vi "SubVI_Overlay Circle Result.vi"(7 "Overlay Result":bool, 8 "Max & min":T2 {"Min Position"."Y" format="%.2f"; "Min Position"."X" format="%.2f"; "Max Position"."Y" format="%.2f"; "Max Position"."X" format="%.2f"}, 9 "Result":cluster{"Name":string, "NG?":bool, "Score":dbl}, 10 "Result In":T3 {"Center"."Y" format="%.2f"; "Center"."X" format="%.2f"}, 11 "Image":T1) -> ()   [LabVIEW 2013]
uses:
  <vilib>/vision/Image Controls.llb/IMAQ Image.ctl
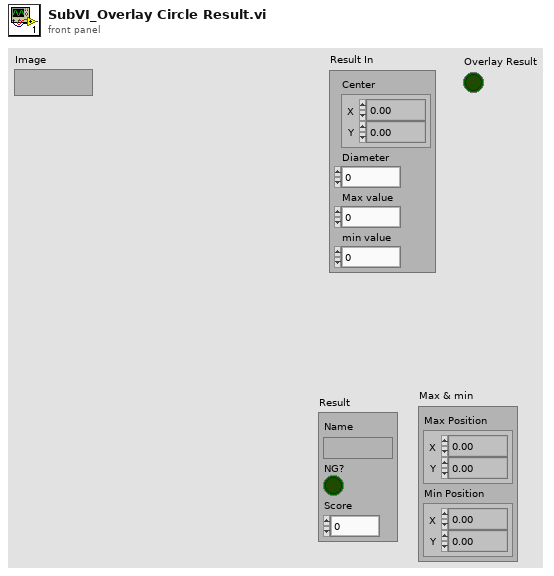
[diagram p1: front panel]
types:
  T1 = typedef "IMAQ Image.ctl" = refnum<image>
  T2 = cluster{"Max Position":cluster{"X":sgl, "Y":sgl}, "Min Position":cluster{"X":sgl, "Y":sgl}}
  T3 = cluster{"Center":cluster{"X":sgl, "Y":sgl}, "Diameter":dbl, "Max value":sgl, "min value":sgl}
  T4 = cluster{"Max Position":cluster{"X":i32, "Y":i32}, "Min Position":cluster{"X":i32, "Y":i32}}
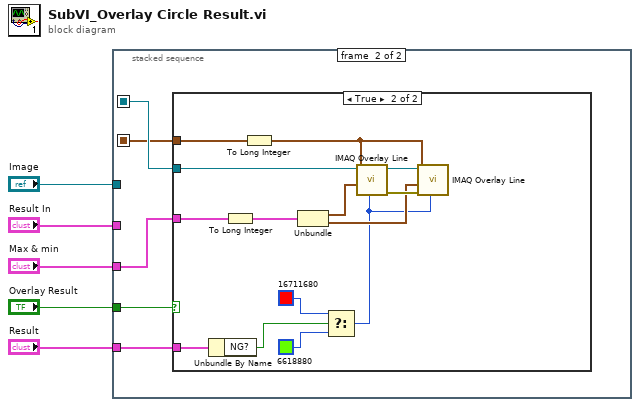
[diagram p0: block diagram]
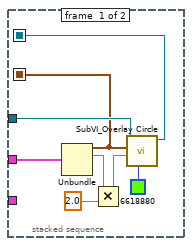
[diagram p2: hidden frame]
diagram:
  n1 = stacked-sequence {
    seq-local: [w10 _] -> [_ w16]
    seq-local: [w9 _] -> [_ w15]
    tunnel: "Image" -> [w11 _]
    tunnel: "Result In" -> [w12 _]
    tunnel: "Max & min" -> [_ w17]
    tunnel: "Overlay Result" -> [_ w18]
    tunnel: "Result" -> [_ w14]
    frame #0 {
      n2 = Unbundle(w12) -> ("Center"=w9:cluster{"X":sgl, "Y":sgl}, "Diameter"=w8:dbl)  [unwired: 2 out]
      n3 = Multiply(x=w8, y=2.0) -> (x*y=w7:dbl)
      n4 = call "SubVI_Overlay Circle.vi"("圓標示顏色"=u32 6618880, "直徑"=w7, "圓心"=w9, "Image"=w11) -> ("Image Out"=w10:T1)  [unwired: 7 in]
    }
    frame #1 {
      n5 = case shown="True" w18 {
        tunnel: w17 -> [_ w27]
        tunnel: w16 -> [_ w25]
        tunnel: w15 -> [_ w24]
        tunnel: w14 -> [_ w23]
        frame False {
        }
        frame True {
          n6 = Unbundle By Name(w23) -> ("NG?"=w22:bool)
          n7 = To Long Integer(number=w27) -> (32bit integer=w26:T4)
          n8 = To Long Integer(number=w24) -> (32bit integer=w31:cluster{"X":i32, "Y":i32})
          n9 = Unbundle(w26) -> ("Max Position"=w28:cluster{"X":i32, "Y":i32}, "Min Position"=w30:cluster{"X":i32, "Y":i32})
          n10 = Select(t=u32 16711680 ("Color"), s=w22, f=u32 6618880 ("Color")) -> (s? t:f=w19:u32)
          n11 = call "IMAQ Overlay Line"("Color"=w19, "End Point"=w28, "Start Point"=w31, "Image"=w25) -> ("error out"=w32:errorcluster, "Image Out"=w29:T1)  [unwired: 6 in]
          n12 = call "IMAQ Overlay Line"("Color"=w19, "error in (no error)"=w32, "End Point"=w30, "Start Point"=w31, "Image"=w29) -> ()  [unwired: 5 in, 2 out]
        }
      }
    }
  }
